vi "Apply Thermocouple Curve.vi"(9 "Internal Temp (°C)":dbl, 11 "TC Reading (°C)":dbl) -> (2 "TC Out (°C)":dbl)   [LabVIEW 2015]
uses:
  <vilib>/Analysis/polynomials.llb/Scalar Polynomial Evaluation (DBL).vi
  <vilib>/Analysis/NI_AALPro.lvlib
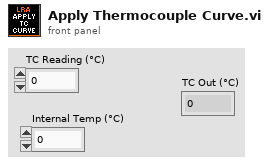
[diagram p1: front panel]
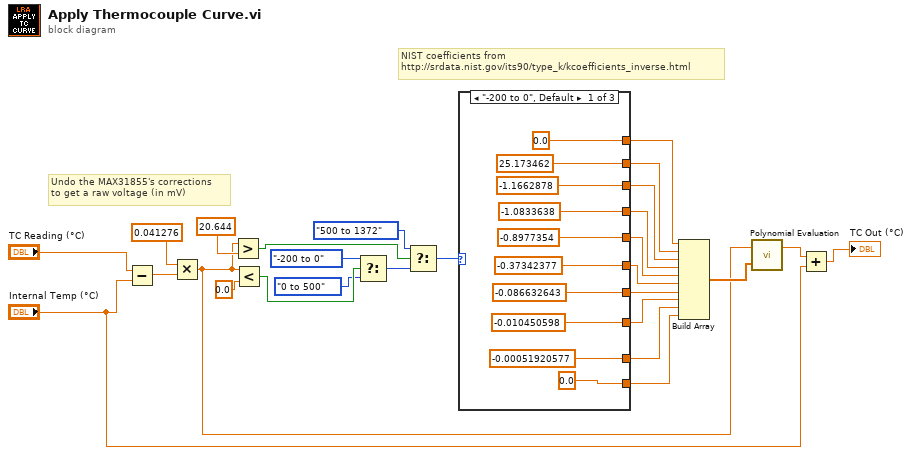
[diagram p0: block diagram]
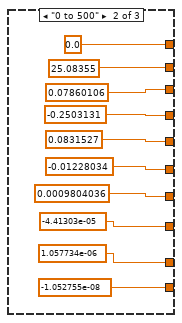
[diagram p2: hidden frame]
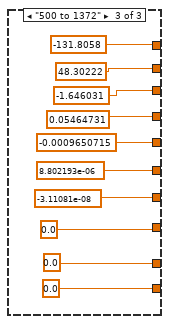
[diagram p3: hidden frame]
diagram:
  # "NIST coefficients from\nhttp://srdata.nist.gov/its90/type_k/kcoefficients_inverse.html"
  # "Undo the MAX31855's corrections\nto get a raw voltage (in mV)"
  n1 = Subtract(x="TC Reading (°C)", y="Internal Temp (°C)") -> (x-y=w26:dbl)
  n2 = Multiply(x=0.041276, y=w26) -> (x*y=w4:dbl)
  n3 = Greater?(x=w4, y=20.644) -> (0:w22:bool)
  n4 = Less?(x=w4, y=0.0) -> (x < y?=w21:bool)
  n5 = Select(t=enum16{"-200 to 0", "0 to 500", "500 to 1372"}."-200 to 0", s=w21, f=enum16{"-200 to 0", "0 to 500", "500 to 1372"}."0 to 500") -> (s? t:f=w20:enum16{"-200 to 0", "0 to 500", "500 to 1372"})
  n6 = Select(t=enum16{"-200 to 0", "0 to 500", "500 to 1372"}."500 to 1372", s=w22, f=w20) -> (s? t:f=w16:enum16{"-200 to 0", "0 to 500", "500 to 1372"})
  n7 = case shown="\"-200 to 0\", Default" w16 {
    tunnel: [0.0 0.0 -131.8058] -> w15
    tunnel: [25.173462 25.08355 48.30222] -> w14
    tunnel: [-1.1662878 0.07860106 -1.646031] -> w13
    tunnel: [-1.0833638 -0.2503131 0.05464731] -> w12
    tunnel: [-0.8977354 0.0831527 -0.0009650715] -> w11
    tunnel: [-0.37342377 -0.01228034 8.802193e-06] -> w10
    tunnel: [-0.086632643 0.0009804036 -3.11081e-08] -> w9
    tunnel: [-0.010450598 -4.41303e-05 0.0] -> w8
    tunnel: [-0.00051920577 1.057734e-06 0.0] -> w7
    tunnel: [0.0 -1.052755e-08 0.0] -> w6
    frame "-200 to 0", Default {
    }
    frame "0 to 500" {
    }
    frame "500 to 1372" {
    }
  }
  n8 = Build Array(w15, w14, w13, w12, w11, w10, w9, w8, w7, w6) -> (w5:dbl[])
  n9 = call-poly <vilib>:"Polynomial Evaluation.vi"("P(x)"=w5, "a"=w4) -> ("P(a)"=w3:dbl)  [unwired: 1 out]
  n10 = Add(x=w3, y="Internal Temp (°C)") -> (x+y=→"TC Out (°C)":dbl)
